vi "get_D.vi"(8 "error in (no error)":errorcluster, 11 "connection ID":refnum<k5>) -> (0 "error out":errorcluster, 2 "D":dbl, 3 "connection ID out":refnum<k5>)   [LabVIEW 2018]
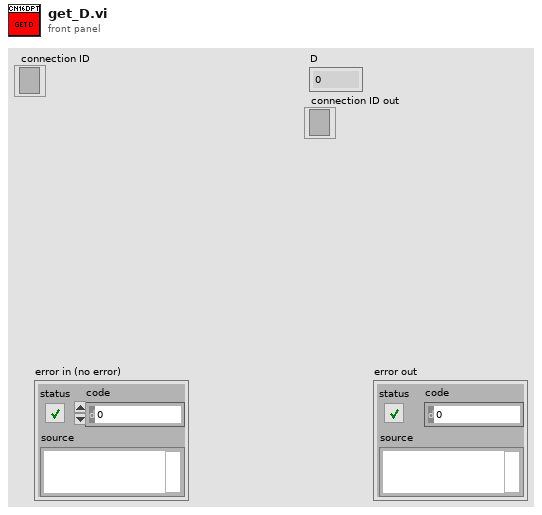
[diagram p1: front panel]
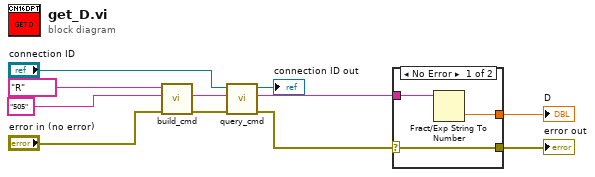
[diagram p0: block diagram]
diagram:
  n1 = call "build_cmd.vi"("error in (no error)"="error in (no error)", "Command ID"="505", "Command class"="R") -> ("error out"=w7:errorcluster, "Command"=w6:string)  [unwired: 7 in]
  n2 = call "query_cmd.vi"("error in (no error)"=w7, "Command"=w6, "connection ID"="connection ID") -> ("error out"=w4:errorcluster, "Response"=w5:string, "connection ID out"=→"connection ID out":refnum<k5>)  [unwired: 6 in]
  n3 = case shown="No Error" w4 {
    selector: w4 -> [w12 w15]
    tunnel: w5 -> [w14 _]
    tunnel: [w12 w15] -> w3
    tunnel: [w13 _] -> w2
    frame No Error {
      n4 = Fract/Exp String To Number(string=w14) -> (number=w13:dbl)  [unwired: 3 in, 1 out]
    }
    frame Error {
    }
  }
  "error out" <- w3
  "D" <- w2
